vi "Log TLS.vi"(8 "error in":errorcluster) -> (0 "error out":errorcluster)   [LabVIEW 2017, in "Akwizycja.lvlib"]
uses:
  Akwizycja.lvlib
panel:
  in  "TLS Cluster":T1
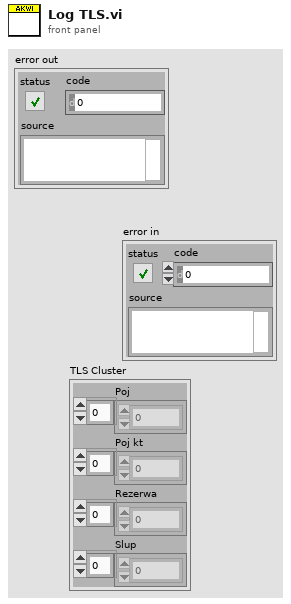
[diagram p1: front panel]
types:
  T1 = cluster{"Poj":sgl[], "Poj kt":sgl[], "Rezerwa":sgl[], "Slup":sgl[]}
  T2 = enum16{"open", "replace", "create", "open or create", "replace or create", "replace or create with confirmation"}
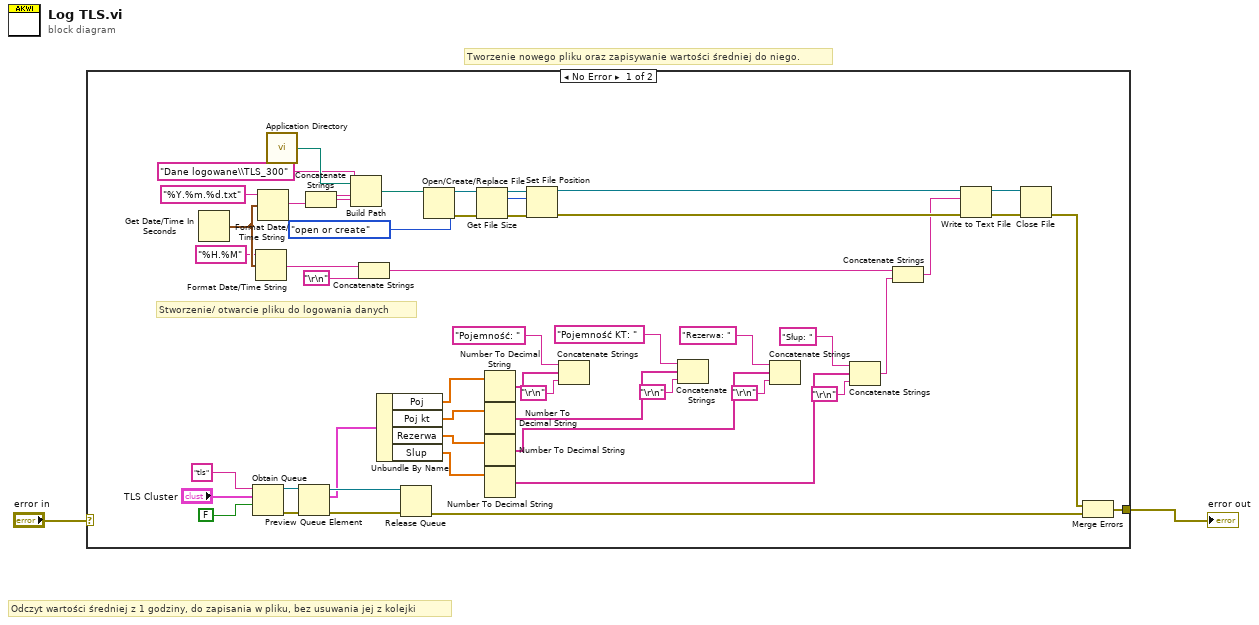
[diagram p0: block diagram]
diagram:
  # "Odczyt wartości średniej z 1 godziny, do zapisania w pliku, bez usuwania jej z kolejki"
  # "Tworzenie nowego pliku oraz zapisywanie wartości średniej do niego."
  n1 = case shown="No Error" "error in" {
    selector: "error in" -> [_ w53]
    tunnel: [w5 w53] -> w1
    frame No Error {
      # "Stworzenie/ otwarcie pliku do logowania danych"
      n2 = Get Date/Time In Seconds() -> (seconds since 1Jan1904=w34:timestamp)
      n3 = Obtain Queue(name (unnamed)="tls", element data type="TLS Cluster", create if not found? (T)=FALSE) -> (queue out=w47:refnum<queue>, error out=w51:errorcluster)  [unwired: 2 in, 1 out]
      n4 = Format Date/Time String(time format string (%c)="%H.%M", seconds (now)=w34) -> (date/time string=w32:string)  [unwired: 1 in]
      n5 = Format Date/Time String(time format string (%c)="%Y.%m.%d.txt", seconds (now)=w34) -> (date/time string=w41:string)  [unwired: 1 in]
      n6 = call <vilib>:"Application Directory.vi"() -> ("Application Directory"=w42:path)
      n7 = Preview Queue Element(queue=w47, error in (no error)=w51) -> (queue out=w50:refnum<queue>, element=w46:T1, error out=w52:errorcluster)  [unwired: 1 in, 1 out]
      n8 = Concatenate Strings("Dane logowane\\TLS_300" ("name or relative path"), w41) -> (w43:string)
      n9 = Build Path(base path=w42, name or relative path=w43) -> (appended path=w44:path)
      n10 = Concatenate Strings(w32, "\r\n") -> (w31:string)
      n11 = Unbundle By Name(w46) -> ("Poj"=w24:sgl[], "Poj kt"=w23:sgl[], "Rezerwa"=w22:sgl[], "Slup"=w21:sgl[])
      n12 = Release Queue(queue=w50, error in (no error)=w52) -> (error out=w6:errorcluster)  [unwired: 1 in, 2 out]
      n13 = Open/Create/Replace File(file path (use dialog)=w44, operation (0:open)=T2."open or create") -> (refnum out=w40:refnum<file>, error out=w39:errorcluster)  [unwired: 4 in, 1 out]
      n14 = Get File Size(file=w40, error in=w39) -> (refnum out=w36:refnum<file>, size (in bytes)=w33:i64, 0:w38:errorcluster)
      n15 = Number To Decimal String(number=w24) -> (decimal integer string=w20:string[])  [unwired: 1 in]
      n16 = Number To Decimal String(number=w23) -> (decimal integer string=w16:string[])  [unwired: 1 in]
      n17 = Number To Decimal String(number=w22) -> (decimal integer string=w11:string[])  [unwired: 1 in]
      n18 = Number To Decimal String(number=w21) -> (decimal integer string=w10:string[])  [unwired: 1 in]
      n19 = Set File Position(offset (in bytes) (0)=w33, refnum=w36, error in=w38) -> (refnum out=w35:refnum<file>, error out=w37:errorcluster)  [unwired: 1 in]
      n20 = Concatenate Strings("Pojemność: " ("string"), w20, "\r\n") -> ()  [unwired: 1 out]
      n21 = Concatenate Strings("Pojemność KT: " ("string"), w16, "\r\n") -> ()  [unwired: 1 out]
      n22 = Concatenate Strings("Rezerwa: " ("string"), w11, "\r\n") -> ()  [unwired: 1 out]
      n23 = Concatenate Strings("Słup: " ("string"), w10, "\r\n") -> (w9:string)
      n24 = Concatenate Strings(w31, w9) -> (w8:string)
      n25 = Write to Text File(file (use dialog)=w35, text=w8, error in=w37) -> (refnum out=w3:refnum<file>, error out=w7:errorcluster)  [unwired: 1 in, 1 out]
      n26 = Close File(refnum=w3, error in=w7) -> (error out=w4:errorcluster)  [unwired: 1 out]
      n27 = Merge Errors(w4, w6) -> (w5:errorcluster)
    }
    frame Error {
    }
  }
  "error out" <- w1
